vi "Initialise globals.vi"(8 "error in (no error)":errorcluster) -> (0 "error out":errorcluster)   [LabVIEW 2017]
uses:
  Peripherals Control/Shutter/Typedefs/Shutter state.ctl
  User Interface/Visualisation/Functional Imaging Viewer/Typedefs/Get-Set-Clear Control.ctl
  Typedefs/Read Write Enum.ctl
  Typedefs/HW config states enum.ctl
  Typedefs/Functional global standard states.ctl
  Typedefs/AVI implementation enum.ctl
  Typedefs/Save-Load enum.ctl
  User Interface/Globals/gl_Windows Ctrl refs.vi
  User Interface/Globals/gl_Funct imaging UI.vi
  General Globals.vi
  Configuration code/Calibration/Globals/gl_Calibration globals.vi
  User Interface/Windows/System config window/Globals/Sys Config window globals.vi
  Peripherals Control/XYZ Stage/Globals/gl_XYZStage globals.vi
  gl_UI Ctrl Refs.vi
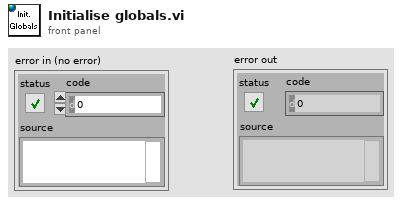
[diagram p1: front panel]
types:
  T1 = typedef "Shutter state.ctl" = enum16{"Closed/Disabled", "Open/Enabled"}
  T2 = enum16{"Initialise", "Load from file", "Save to file", "Read", "Write"}
  T3 = typedef "Functional global standard states.ctl" = enum16{"Initialise", "Read", "Write", "Load", "Save", "Clear"}
  T4 = typedef "Read Write Enum.ctl" = enum16{"Read", "Write"}
  T5 = typedef "Get-Set-Clear Control.ctl" = enum16{"Get", "Set", "Clear"}
  T6 = typedef "Save-Load enum.ctl" = enum16{"Save to file", "Load from file", "Compare from file"}
  T7 = typedef "AVI implementation enum.ctl" = enum16{"AVI1", "AVI2"}
  T8 = enum16{"Write Red AVI", "Write Green AVI", "Write AVI mode"}[]
  T9 = typedef "HW config states enum.ctl" = enum16{"Load from file", "Save to file", "Write all", "Read all", "Write XY stage settings", "Write DAQ FPGA settings", "Write Control FPGA settings", "Write Phys Channels", "Write System Config", "Write HW Config", "Save System Config", "Save HW Config", "Clear", "Compare from file"}
  T10 = typedef "Calibration config.ctl" = cluster{"Current Objective":string, "Objective Settings":T11[], "PreChirper Values Preset ?":bool, "PreChirper Settings":T12[], "PreChirper Constants":T13}
  T11 = typedef "Objective Config.ctl" = cluster{"Name":string, "Sum X":dbl, "Sum Y":dbl, "Diff X":dbl, "Diff Y":dbl, "Distortion Correction":dbl, "Z_norm to um_scaling":dbl, "X_norm to um_scaling":dbl, "Calibrated Wavelength":dbl}
  T12 = typedef "Prechirper Cal Config.ctl" = cluster{"Wavelength":i32, "Prism 1":i32, "Prism 2":i32}
  T13 = typedef "PreChirper constants.ctl" = cluster{"a 1":i32, "b 1":i32, "c 1":i32, "a 2":i32, "b 2":i32, "c 2":i32, "lmin":i32, "lmax":i32}
  T14 = typedef "UI ctrl refs cluster.ctl" = cluster{"Top level VI path":path, "Top level VI ref":refnum<vi>, "User menu ref":refnum<k9>, "Sub Panel control":refnum<vi>, "Imaging Param Tab":refnum<vi>, "Occurrence-Start drivers":refnum<k4>, "Occurrence-Speed logging initialised":refnum<k4>, "Occurrence-XYZ stage initialised":refnum<k4>, "Exit button":refnum<vi>, "Status ind":refnum<vi>, "Set as origin":refnum<vi>, "Speed Logging":refnum<vi>, "Time Lapse":refnum<vi>, "Live Imaging":refnum<vi>, "AOL Z Stack":refnum<vi>, "Motor Z Stack":refnum<vi>, "Funct Acq button":refnum<vi>, "Hard Shutter":refnum<vi>, "Virtual Shutter":refnum<vi>, "Laser Power":refnum<vi>, "AOL Mode":refnum<vi>, "Frame Size":refnum<vi>, "Field of View":refnum<vi>, "Dwell Time":refnum<vi>, "Zoom":refnum<vi>, "AOL Z":refnum<vi>, "Objective":refnum<vi>, "Axis":refnum<vi>, "Paths & Names":refnum<vi>, "Experiment folder path (ind.)":refnum<vi>, "Last State (Ind.)":refnum<vi>, "Averages":refnum<vi>, "Angle (degrees)":refnum<vi>, "X centre":refnum<vi>, "Y centre":refnum<vi>, "Plane Mode":refnum<vi>, "# Planes":refnum<vi>, "Z Start":refnum<vi>, "Z Stop":refnum<vi>, "Z Step":refnum<vi>, "PMT 1":refnum<vi>, "PMT 2":refnum<vi>, "Stage XYZ Position":refnum<vi>, "Pockels@Z Start":refnum<vi>, "Pockels@Z Stop":refnum<vi>, "Obtain Z Start":refnum<vi>, "Obtain Z Stop":refnum<vi>, "Live stim.trig.period":refnum<vi>, "Live stim.trig.enable":refnum<vi>, "Funct. Acq. Pockels Modulation":refnum<vi>, "Enable Video Recording":refnum<vi>, "Video Record-Live Imaging":refnum<vi>, "Video Record-Funct acq":refnum<vi>, "AOL Z-stack Chirps Ready (ind)":refnum<vi>, "Center freq ind (nm)":refnum<vi>, "Logging queue (ind)":refnum<vi>, "Back aperture power (ind.)":refnum<vi>, "Power after objective (ind.)":refnum<vi>, "Switch user":refnum<vi>, "Ls1 Conn. Status":refnum<vi>, "Ls1Tuning Status":refnum<vi>, "Ls1 Faults":refnum<vi>, "Ls1 Connection":refnum<vi>, "Ls1 Mode":refnum<vi>, "Ls1 POWER [mW]":refnum<vi>, "Ls1Shutter":refnum<vi>, "Ls1 Wavelength":refnum<vi>, "Ls1 Note":refnum<vi>, "Ls1 Confirm Wav":refnum<vi>, "Ls1 PreChrp Prism1":refnum<vi>, "Ls1 PreChrp Prism2":refnum<vi>, "Ls1 wav top Ind":refnum<vi>, "Ls1 power top Ind":refnum<vi>, "Ls1 Pump peak Hold":refnum<vi>, "Ls1 Status Ind":refnum<vi>, "Ls1 wav cancel":refnum<vi>, "Experiment Type":refnum<vi>, "Biology Information":refnum<vi>}
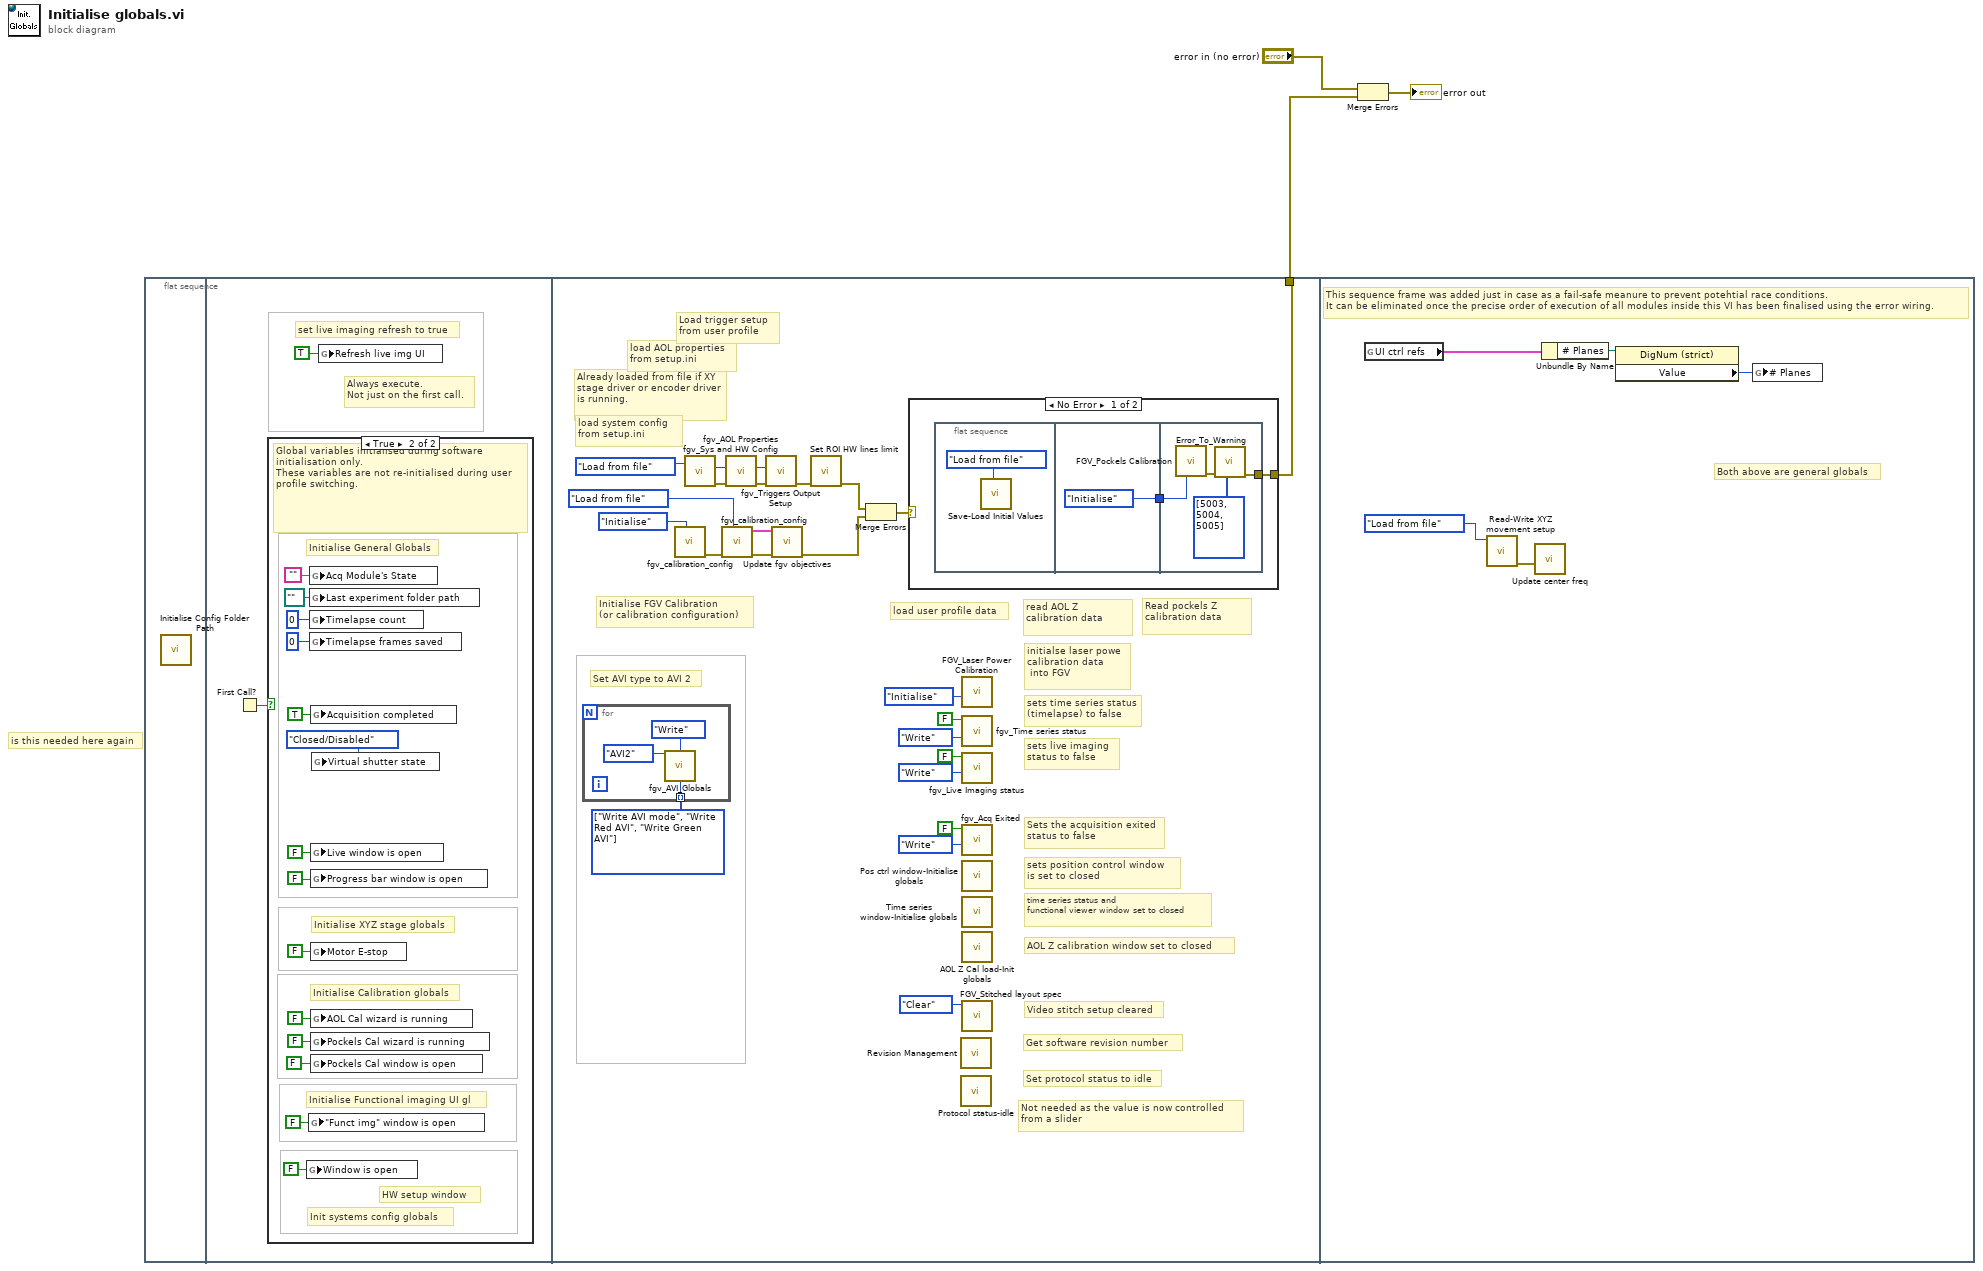
[diagram p0: block diagram]
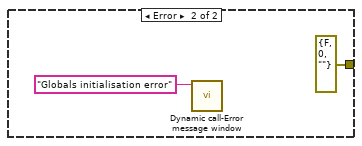
[diagram p3: hidden frame]
diagram:
  # "is this needed here again"
  n1 = flat-sequence {
    tunnel: [w31] -> w3
    frame #0 {
      n2 = call "Initialise Config Folder Path.vi"() -> ()  [unwired: 9 in, 3 out]
    }
    frame #1 {
      # "set live imaging refresh to true"
      # "Always execute.\nNot just on the first call."
      n3 = First Call?() -> (First Call?: T/F=w5:bool)
      n4 = case shown="True" w5 {
        frame False {
        }
        frame True {
          # "Init systems config globals"
          # "Initialise Functional imaging UI gl"
          # "Initialise Calibration globals"
          # "Initialise XYZ stage globals"
          # "Initialise General Globals"
          # "HW setup window"
          # "Global variables initialised during software initialisation only.\nThese variables are not re-initialised during user profile switching."
          n5 = global write "Sys Config window globals.vi" "Window is open"(FALSE ("Bring to front")) -> ()
          n6 = global write "gl_Funct imaging UI.vi" "\"Funct img\" window is open"(FALSE ("\"Funct img\" window is open")) -> ()
          n7 = global write "General Globals.vi" "Acq Module's State"("" ("Acq Module's State")) -> ()
          n8 = global write "General Globals.vi" "Last experiment folder path"(path "" ("Last experiment folder path")) -> ()
          n9 = global write "General Globals.vi" "Timelapse count"(u32 0 ("Timelapse count")) -> ()
          n10 = global write "General Globals.vi" "Timelapse frames saved"(u32 0 ("Timelapse frames saved")) -> ()
          n11 = global write "General Globals.vi" "Acquisition completed"(TRUE ("Acquisition completed")) -> ()
          n12 = global write "General Globals.vi" "Live window is open"(FALSE ("Live window running")) -> ()
          n13 = global write "General Globals.vi" "Progress bar window is open"(FALSE ("Progress bar window is open")) -> ()
          n14 = global write "gl_XYZStage globals.vi" "Motor E-stop"(FALSE ("Motor E-stop")) -> ()
          n15 = global write "gl_Calibration globals.vi" "AOL Cal wizard is running"(FALSE ("Motor Z Cal wizard is running")) -> ()
          n16 = global write "gl_Calibration globals.vi" "Pockels Cal wizard is running"(FALSE ("Pockels Cal wizard is running")) -> ()
          n17 = global write "gl_Calibration globals.vi" "Pockels Cal window is open"(FALSE ("Pockels Cal window is open")) -> ()
          n18 = global write "General Globals.vi" "Virtual shutter state"(Shutter_state."Closed/Disabled" ("Virtual shutter state")) -> ()
        }
      }
      n19 = global write "gl_Windows Ctrl refs.vi" "Refresh live img UI"(TRUE ("Refresh live img UI")) -> ()
    }
    frame #2 {
      w34 = T8 [enum."Write AVI mode", enum."Write Red AVI", enum."Write Green AVI"] items=["Write Red AVI", "Write Green AVI", "Write AVI mode"]
      w30 = HW_config_states_enum."Load from file" ("Function")
      # "Not needed as the value is now controlled\nfrom a slider"
      # "Initialise FGV Calibration\n(or calibration configuration)"
      # "Set protocol status to idle"
      # "Get software revision number"
      # "Video stitch setup cleared"
      # "AOL Z calibration window set to closed"
      # "time series status and \nfunctional viewer window set to closed"
      # "sets position control window\nis set to closed"
      # "Sets the acquisition exited\nstatus to false"
      # "sets live imaging \nstatus to false"
      # "sets time series status\n(timelapse) to false"
      # "initialse laser powe \ncalibration data\n into FGV"
      # "Set AVI type to AVI 2"
      # "Read pockels Z calibration data"
      # "read AOL Z calibration data"
      # "load user profile data"
      # "Load trigger setup \nfrom user profile"
      # "load AOL properties\nfrom setup.ini"
      # "load system config \nfrom setup.ini"
      # "Already loaded from file if XY stage driver or encoder driver is running."
      n20 = for {
        tunnel: w34 -> [w52] mode=indexing
        n21 = call "fgv_AVI_Globals.vi"("AVI mode"=AVI_implementation_enum."AVI2", "Function"=enum16{"Intialize", "Write", "Read", "Clear"}."Write", "\"Write\" sub function"=w52) -> ()  [unwired: 9 in, 4 out]
      }
      n22 = call "fgv_calibration_config.vi"("Cal config ops"=T2."Initialise") -> ("error out"=w27:errorcluster)  [unwired: 9 in, 1 out]
      n23 = call "fgv_Sys and HW Config.vi"("Function"=w30) -> ("error out"=w33:errorcluster)  [unwired: 8 in, 2 out]
      n24 = call "fgv_calibration_config.vi"("Cal config ops"=T2."Load from file", "error in (no error)"=w27) -> ("error out"=w24:errorcluster, "Config cluster OUT"=w22:T10)  [unwired: 8 in]
      n25 = call "fgv_AOL Properties.vi"("error in (no error)"=w33, "Function"=w30) -> ("error out"=w32:errorcluster)  [unwired: 8 in, 1 out]
      n26 = call "fgv_Triggers Output Setup.vi"("error in (no error)"=w32, "Function"=w30) -> ("error out"=w21:errorcluster)  [unwired: 7 in, 2 out]
      n27 = call "Update fgv objectives.vi"("error in (no error)"=w24, "Config cluster IN"=w22) -> ("error out"=w23:errorcluster)  [unwired: 9 in]
      n28 = call "Set ROI HW lines limit.vi"("error in (no error)"=w21) -> ("error out"=w20:errorcluster)  [unwired: 10 in]
      n29 = Merge Errors(w20, w23) -> (w25:errorcluster)
      n30 = case shown="No Error" w25 {
        tunnel: [w43 errorcluster {"status"=FALSE, "code"=0, "source"=""} ("error out")] -> w31
        frame No Error {
          n31 = flat-sequence {
            tunnel: [Functional_global_standard_states."Initialise" ("Function")] -> w42
            tunnel: [w47] -> w43
            tunnel: w42 -> [w46]
            frame #0 {
              n32 = call "Save-Load Initial Values.vi"("Function"=Save-Load_enum."Load from file") -> ()  [unwired: 10 in, 1 out]
            }
            frame #1 {
            }
            frame #2 {
              n33 = call "FGV_Pockels Calibration.vi"("Function"=w46) -> ("error out"=w49:errorcluster)  [unwired: 4 in, 6 out]
              n34 = call <userlib>:"Error_To_Warning.vi"("Error Codes to be handled as warnings"=i32[] [5003, 5004, 5005], "error in"=w49) -> ("error out"=w47:errorcluster)  [unwired: 9 in]
            }
          }
        }
        frame Error {
          n35 = call "Dynamic call-Error message window.vi"("Error Message"="Globals initialisation error" ("message")) -> ()  [unwired: 10 in, 1 out]
        }
      }
      n36 = call "Revision Management.vi"() -> ()  [unwired: 11 in, 1 out]
      n37 = call "Protocol status-idle.vi"() -> ()  [unwired: 12 in]
      n38 = call "FGV_Laser Power Calibration.vi"("Function"=Functional_global_standard_states."Initialise") -> ()  [unwired: 7 in, 4 out]
      n39 = call "fgv_Time series status.vi"("Function"=Read_Write_Enum."Write", "Timelapse?"=FALSE) -> ()  [unwired: 9 in, 1 out]
      n40 = call "fgv_Live Imaging status.vi"("Function"=Read_Write_Enum."Write", "Live Imaging?"=FALSE) -> ()  [unwired: 8 in, 2 out]
      n41 = call "fgv_Acq Exited.vi"("Function"=Read_Write_Enum."Write", "Acquisition completed"=FALSE ("Timelapse?")) -> ()  [unwired: 8 in, 2 out]
      n42 = call "Pos ctrl window-Initialise globals.vi"() -> ()  [unwired: 12 in]
      n43 = call "Time series window-Initialise globals.vi"() -> ()  [unwired: 12 in]
      n44 = call "AOL Z Cal load-Init globals.vi"() -> ()  [unwired: 12 in]
      n45 = call "FGV_Stitched layout spec.vi"("Function"=Get-Set-Clear_Control."Clear") -> ()  [unwired: 9 in, 2 out]
    }
    frame #3 {
      # "Both above are general globals"
      # "This sequence frame was added just in case as a fail-safe meanure to prevent potehtial race conditions.\nIt can be eliminated once the precise order of execution of all modules inside this VI has been finalised using the error wiring."
      n46 = global read "gl_UI Ctrl Refs.vi" "UI ctrl refs"() -> (w57:T14)
      n47 = call "Read-Write XYZ movement setup.vi"("Function"=Save-Load_enum."Load from file") -> ("error out"=w55:errorcluster)  [unwired: 10 in]
      n48 = call "Update center freq.vi"("error in (no error)"=w55) -> ()  [unwired: 10 in, 1 out]
      n49 = Unbundle By Name(w57) -> ("# Planes"=w59:refnum<vi>)
      n50 = property class="DigNum (strict)"(reference=w59) -> ("Value"=w58:u16)  [unwired: 1 in, 2 out]
      n51 = global write "General Globals.vi" "# Planes"(w58) -> ()
    }
  }
  n52 = Merge Errors("error in (no error)", w3) -> (→"error out":errorcluster)
